vi "retirar NaN.vi"(11 "Array":T1(array[cluster])) -> (3 "Array Out":T1(array[cluster]))   [LabVIEW 2016]
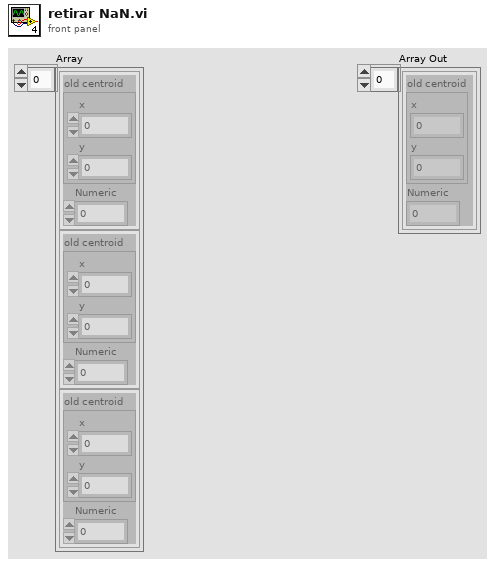
[diagram p1: front panel]
types:
  T1 = cluster{"old centroid":cluster{"x":dbl, "y":dbl}, "Numeric":i32}[]
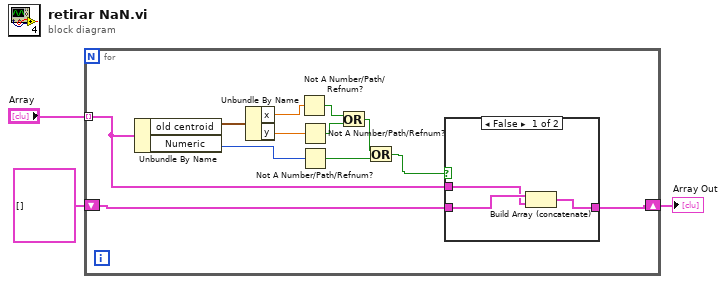
[diagram p0: block diagram]
diagram:
  n1 = for {
    tunnel: "Array" -> [w4] mode=indexing
    shift-right: [w6] -> w1
    shift-left: T1 [] -> [w7]
    n2 = Unbundle By Name(w4) -> ("old centroid"=w11:cluster{"x":dbl, "y":dbl}, "Numeric"=w8:i32)
    n3 = Unbundle By Name(w11) -> ("x"=w10:dbl, "y"=w9:dbl)
    n4 = Not A Number/Path/Refnum?(number/path/refnum=w10) -> (NaN/Path/Refnum?=w15:bool)
    n5 = Not A Number/Path/Refnum?(number/path/refnum=w9) -> (NaN/Path/Refnum?=w14:bool)
    n6 = Not A Number/Path/Refnum?(number/path/refnum=w8) -> (NaN/Path/Refnum?=w12:bool)
    n7 = Or(x=w15, y=w14) -> (x .or. y?=w13:bool)
    n8 = Or(x=w13, y=w12) -> (x .or. y?=w5:bool)
    n9 = case shown="False" w5 {
      tunnel: w7 -> [w18 w19]
      tunnel: [w17 w19] -> w6
      tunnel: w4 -> [w16 _]
      frame False {
        n10 = Build Array (concatenate)(w18, w16) -> (w17:T1)
      }
      frame True {
      }
    }
  }
  "Array Out" <- w1
